vi "subJoystick.vi"(1 "Index":i32=1) -> ()   [LabVIEW 2020]
panel:
  out "AxisZ":i32
  in  "joy button":bool caption="evaluate joystick button"
  in  "Save":bool
  in  "Zone":u32 max=256
  in  "Zzero":u32 caption="Z-Null" max=1023
  in  "Yzero":u32 caption="Y-Null" max=1023
  in  "Xzero":u32 caption="X-Null" max=1023
  in  "SetAcc":bool
  in  "AccZ":i32 caption="Z" min=0
  in  "AccY":i32 caption="Y" min=0
  in  "VelZ":dbl caption="Z, [Hz]" step=0.1 format="%.3f"
  in  "VelY":dbl caption="Y, [Hz]" step=0.1 format="%.3f"
  in  "z3":bool caption="3"
  in  "z2":bool caption="2"
  in  "z1":bool caption="1"
  out "RAcc":bool
  out "RVel":bool
  out "AxisY":i32
  out "AxisX":i32
  in  "AccX":i32 caption="X" min=0
  in  "VelX":dbl caption="X, [Hz]" step=0.1 format="%.3f"
  in  "SetVel":bool
  in  "y3":bool caption="3"
  in  "y2":bool caption="2"
  in  "y1":bool caption="1"
  in  "x3":bool caption="3"
  in  "x2":bool caption="2"
  in  "x1":bool caption="1"
  in  "Set":bool
  in  "Close":bool
  # "Axis X"
  # "Axis Y"
  # "Axis Z"
  # "Joystick speed"
  # "Joystick acceleration"
  # "Joystick settings"
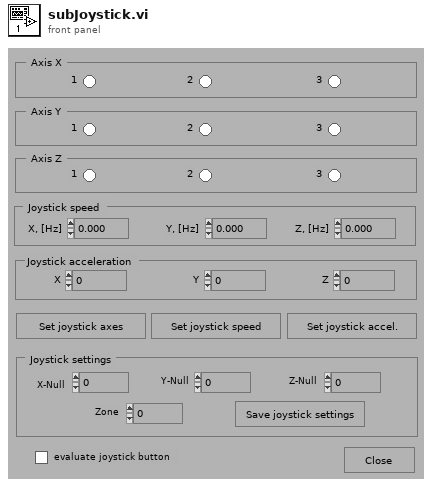
[diagram p1: front panel]
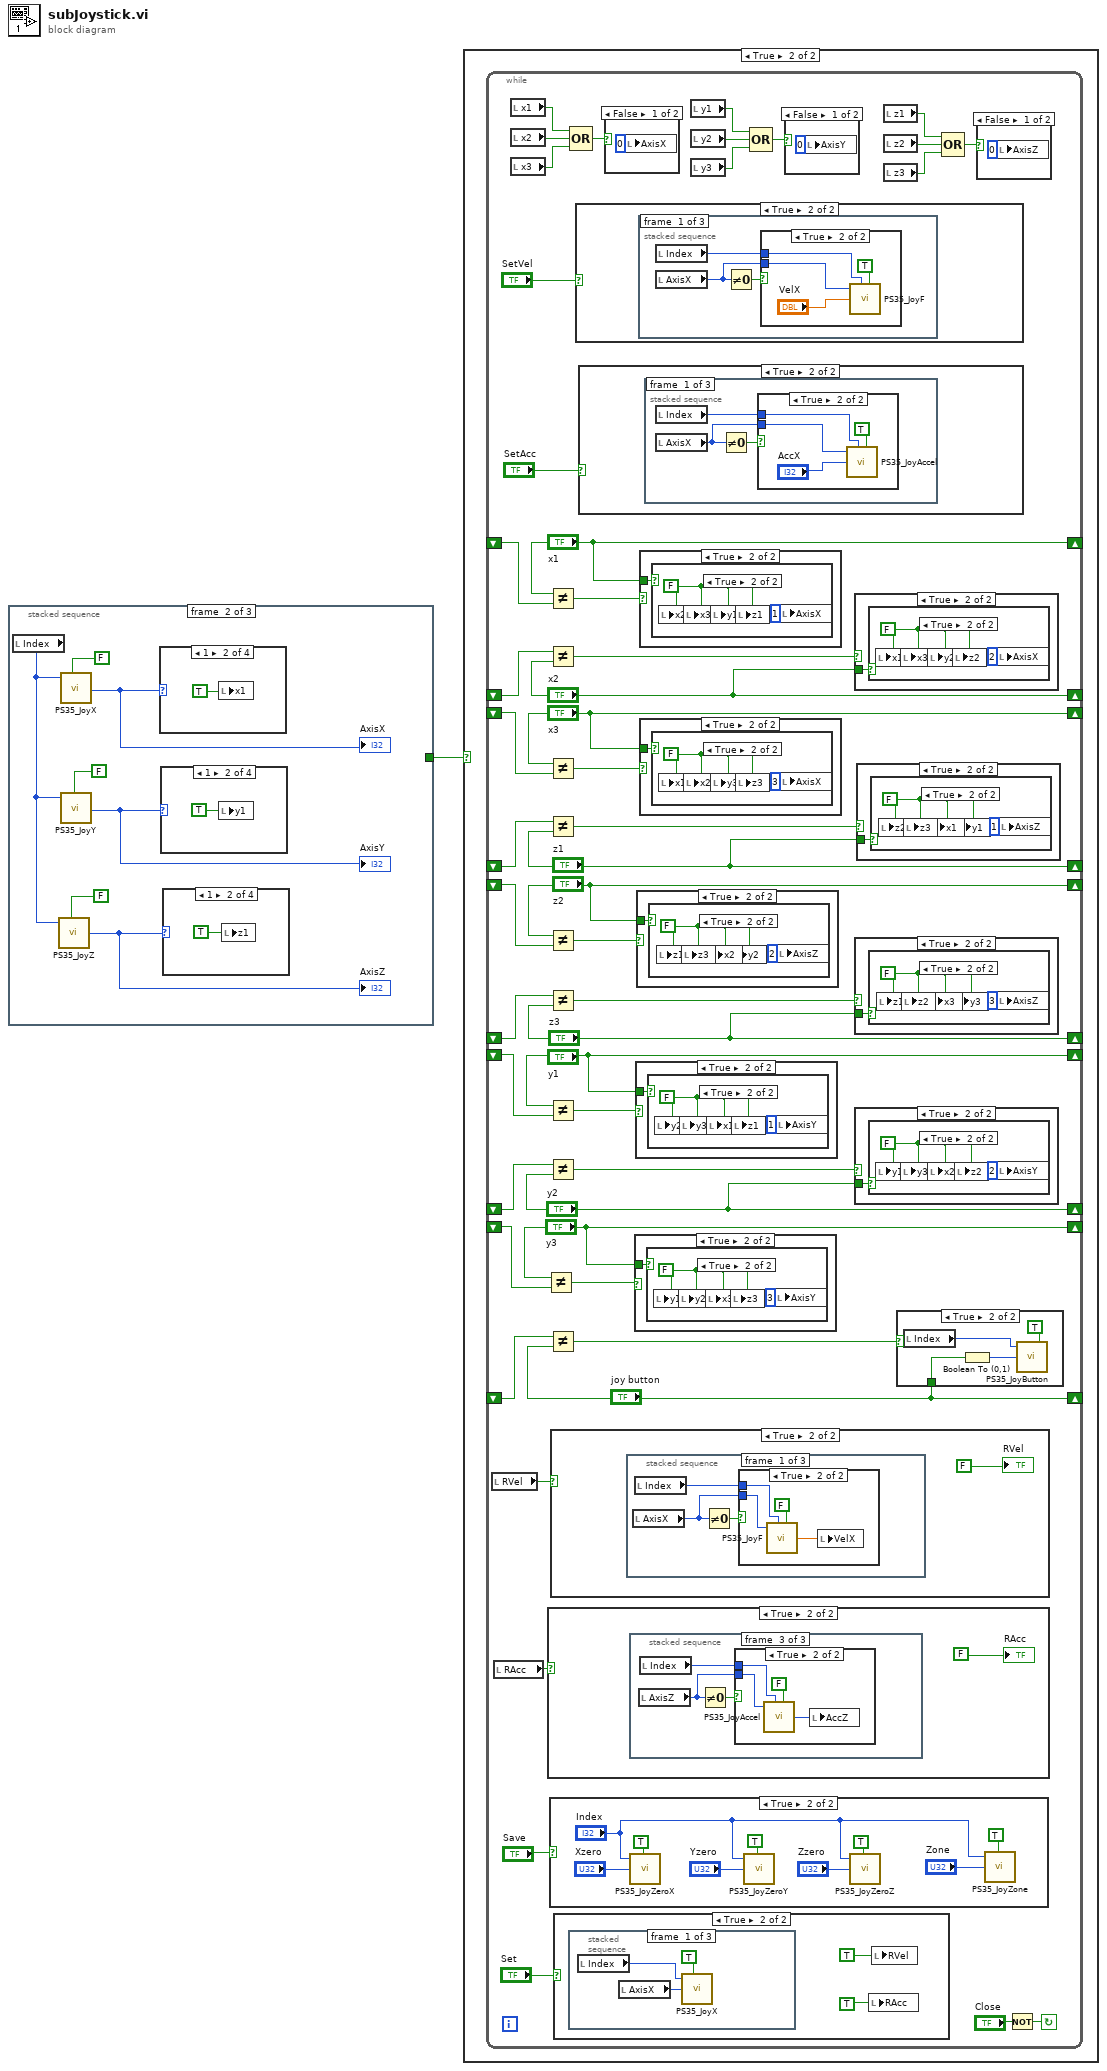
[diagram p0: block diagram]
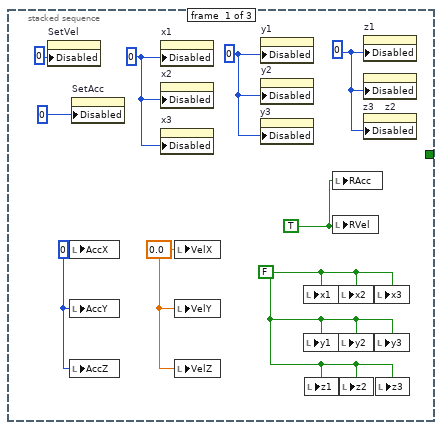
[diagram p2: hidden frame]
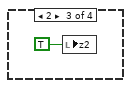
[diagram p4: hidden frame]
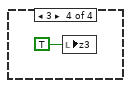
[diagram p5: hidden frame]
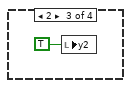
[diagram p7: hidden frame]
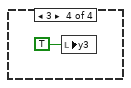
[diagram p8: hidden frame]
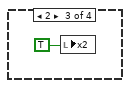
[diagram p10: hidden frame]
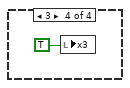
[diagram p11: hidden frame]
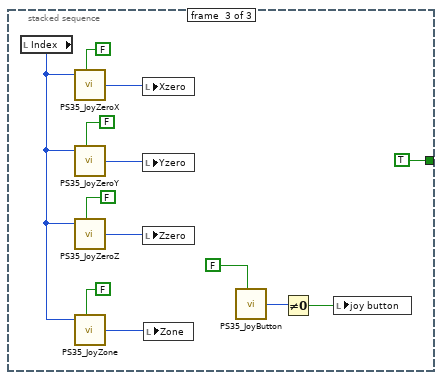
[diagram p12: hidden frame]
diagram:
  n1 = stacked-sequence {
    tunnel: [_ _ TRUE] -> w1
    frame #0 {
      w2 = 0.0 ("VelX")
      w3 = 0 ("AccX")
      w4 = FALSE ("WriteRead")
      w5 = TRUE
      w6 = u8 0 ("Disabled")
      w7 = u8 0 ("Disabled")
      w8 = u8 0 ("Disabled")
      n2 = property on="SetVel" class="Bool"("Disabled"=u8 0) -> ()  [unwired: 2 in, 2 out]
      n3 = local write "AccX"(w3) -> ()
      n4 = local write "AccY"(w3) -> ()
      n5 = local write "AccZ"(w3) -> ()
      n6 = property on="SetAcc" class="Bool"("Disabled"=0 ("Nr")) -> ()  [unwired: 2 in, 2 out]
      n7 = property on="x1" class="Bool (strict)"("Disabled"=w8) -> ()  [unwired: 2 in, 2 out]
      n8 = property on="x2" class="Bool (strict)"("Disabled"=w8) -> ()  [unwired: 2 in, 2 out]
      n9 = property on="x3" class="Bool (strict)"("Disabled"=w8) -> ()  [unwired: 2 in, 2 out]
      n10 = local write "VelX"(w2) -> ()
      n11 = local write "VelY"(w2) -> ()
      n12 = local write "VelZ"(w2) -> ()
      n13 = property on="y1" class="Bool (strict)"("Disabled"=w7) -> ()  [unwired: 2 in, 2 out]
      n14 = property on="y2" class="Bool (strict)"("Disabled"=w7) -> ()  [unwired: 2 in, 2 out]
      n15 = property on="y3" class="Bool (strict)"("Disabled"=w7) -> ()  [unwired: 2 in, 2 out]
      n16 = local write "x1"(w4) -> ()
      n17 = local write "y1"(w4) -> ()
      n18 = local write "z1"(w4) -> ()
      n19 = local write "RAcc"(w5) -> ()
      n20 = local write "RVel"(w5) -> ()
      n21 = local write "x2"(w4) -> ()
      n22 = local write "y2"(w4) -> ()
      n23 = local write "z2"(w4) -> ()
      n24 = property on="z1" class="Bool (strict)"("Disabled"=w6) -> ()  [unwired: 2 in, 2 out]
      n25 = property on="z2" class="Bool (strict)"("Disabled"=w6) -> ()  [unwired: 2 in, 2 out]
      n26 = property on="z3" class="Bool (strict)"("Disabled"=w6) -> ()  [unwired: 2 in, 2 out]
      n27 = local write "x3"(w4) -> ()
      n28 = local write "y3"(w4) -> ()
      n29 = local write "z3"(w4) -> ()
    }
    frame #1 {
      n30 = local read "Index"() -> (w11:i32)
      n31 = call "PS35_JoyZ.vi"("Control unit ID"=w11, "function"=FALSE) -> ("Value-Out"=w12:i32)  [unwired: 6 in, 1 out]
      "AxisZ" <- w12
      n32 = call "PS35_JoyX.vi"("Control unit ID"=w11, "function"=FALSE) -> ("Value-Out"=w14:i32)  [unwired: 6 in, 1 out]
      "AxisX" <- w14
      n33 = call "PS35_JoyY.vi"("Control unit ID"=w11, "function"=FALSE) -> ("Value-Out"=w13:i32)  [unwired: 6 in, 1 out]
      "AxisY" <- w13
      n34 = case shown="1" w14 {
        frame 0, Default {
        }
        frame 1 {
          n35 = local write "x1"(TRUE ("WriteRead")) -> ()
        }
        frame 2 {
          n36 = local write "x2"(TRUE ("WriteRead")) -> ()
        }
        frame 3 {
          n37 = local write "x3"(TRUE ("WriteRead")) -> ()
        }
      }
      n38 = case shown="1" w13 {
        frame 0, Default {
        }
        frame 1 {
          n39 = local write "y1"(TRUE ("y1")) -> ()
        }
        frame 2 {
          n40 = local write "y2"(TRUE ("y1")) -> ()
        }
        frame 3 {
          n41 = local write "y3"(TRUE ("y1")) -> ()
        }
      }
      n42 = case shown="1" w12 {
        frame 0, Default {
        }
        frame 1 {
          n43 = local write "z1"(TRUE ("y1")) -> ()
        }
        frame 2 {
          n44 = local write "z2"(TRUE ("y1")) -> ()
        }
        frame 3 {
          n45 = local write "z3"(TRUE ("y1")) -> ()
        }
      }
    }
    frame #2 {
      n46 = local read "Index"() -> (w27:i32)
      n47 = call "PS35_JoyZeroX.vi"("Control unit ID"=w27, "function"=FALSE) -> ("Value-Out"=w37:i32)  [unwired: 6 in, 1 out]
      n48 = call "PS35_JoyZeroY.vi"("Control unit ID"=w27, "function"=FALSE) -> ("Value-Out"=w36:i32)  [unwired: 6 in, 1 out]
      n49 = call "PS35_JoyZeroZ.vi"("Control unit ID"=w27, "function"=FALSE) -> ("Value-Out"=w33:i32)  [unwired: 6 in, 1 out]
      n50 = call "PS35_JoyZone.vi"("Control unit ID"=w27, "function"=FALSE) -> ("Value-Out"=w32:i32)  [unwired: 6 in, 1 out]
      n51 = local write "Xzero"(w37) -> ()
      n52 = local write "Yzero"(w36) -> ()
      n53 = local write "Zzero"(w33) -> ()
      n54 = local write "Zone"(w32) -> ()
      n55 = call "PS35_JoyButton.vi"("function"=FALSE) -> ("Value-Out"=w29:i32)  [unwired: 7 in, 1 out]
      n56 = Not Equal To 0?(x=w29) -> (x != 0?=w28:bool)
      n57 = local write "joy button"(w28) -> ()
    }
  }
  n58 = case shown="True" w1 {
    frame False {
    }
    frame True {
      n59 = while {
        shift-left: _ -> [w77]
        shift-right: ["joy button"] -> _
        shift-left: _ -> [w79]
        shift-right: ["y3"] -> _
        shift-left: _ -> [w81]
        shift-right: ["y2"] -> _
        shift-left: _ -> [w80]
        shift-right: ["y1"] -> _
        shift-left: _ -> [w82]
        shift-right: ["z3"] -> _
        shift-left: _ -> [w83]
        shift-right: ["z2"] -> _
        shift-left: _ -> [w85]
        shift-right: ["z1"] -> _
        shift-left: _ -> [w84]
        shift-right: ["x3"] -> _
        shift-left: _ -> [w86]
        shift-right: ["x2"] -> _
        shift-left: _ -> [w87]
        shift-right: ["x1"] -> _
        stop <- w89 continue-if-true
        n60 = local read "RVel"() -> (w72:bool)
        n61 = local read "RAcc"() -> (w71:bool)
        n62 = local read "x1"() -> (w50:bool)
        n63 = local read "x2"() -> (w51:bool)
        n64 = local read "x3"() -> (w49:bool)
        n65 = Not Equal?(x="y3", y=w79) -> (x != y?=w53:bool)
        n66 = Not Equal?(x="x1", y=w87) -> (x != y?=w69:bool)
        n67 = Not Equal?(x=w86, y="x2") -> (x != y?=w67:bool)
        n68 = Not Equal?(x="x3", y=w84) -> (x != y?=w65:bool)
        n69 = Not Equal?(x=w85, y="z1") -> (x != y?=w63:bool)
        n70 = Not Equal?(x="z2", y=w83) -> (x != y?=w61:bool)
        n71 = Not Equal?(x=w82, y="z3") -> (x != y?=w59:bool)
        n72 = Not Equal?(x="y1", y=w80) -> (x != y?=w57:bool)
        n73 = Not Equal?(x=w81, y="y2") -> (x != y?=w55:bool)
        n74 = Not Equal?(x=w77, y="joy button") -> (x != y?=w75:bool)
        n75 = case shown="True" w71 {
          frame False {
          }
          frame True {
            n76 = stacked-sequence {
              frame #0 {
                n77 = local read "Index"() -> (w127:i32)
                n78 = local read "AxisX"() -> (w129:i32)
                n79 = Not Equal To 0?(x=w129) -> (x != 0?=w128:bool)
                n80 = case shown="True" w128 {
                  tunnel: w129 -> [_ w133]
                  tunnel: w127 -> [_ w131]
                  frame False {
                    n81 = local write "AccX"(0 ("AccX")) -> ()
                  }
                  frame True {
                    n82 = call "PS35_JoyAccel.vi"("Axis number"=w133, "Control unit ID"=w131, "function"=FALSE ("WriteRead")) -> ("Value-Out"=w132:i32)  [unwired: 5 in, 1 out]
                    n83 = local write "AccX"(w132) -> ()
                  }
                }
              }
              frame #1 {
                n84 = local read "AxisY"() -> (w137:i32)
                n85 = local read "Index"() -> (w135:i32)
                n86 = Not Equal To 0?(x=w137) -> (x != 0?=w136:bool)
                n87 = case shown="True" w136 {
                  tunnel: w137 -> [_ w141]
                  tunnel: w135 -> [_ w139]
                  frame False {
                    n88 = local write "AccY"(0 ("AccX")) -> ()
                  }
                  frame True {
                    n89 = call "PS35_JoyAccel.vi"("Axis number"=w141, "Control unit ID"=w139, "function"=FALSE ("WriteRead")) -> ("Value-Out"=w140:i32)  [unwired: 5 in, 1 out]
                    n90 = local write "AccY"(w140) -> ()
                  }
                }
              }
              frame #2 {
                n91 = local read "AxisZ"() -> (w145:i32)
                n92 = local read "Index"() -> (w143:i32)
                n93 = Not Equal To 0?(x=w145) -> (x != 0?=w144:bool)
                n94 = case shown="True" w144 {
                  tunnel: w145 -> [_ w149]
                  tunnel: w143 -> [_ w147]
                  frame False {
                    n95 = local write "AccZ"(0 ("AccX")) -> ()
                  }
                  frame True {
                    n96 = call "PS35_JoyAccel.vi"("Axis number"=w149, "Control unit ID"=w147, "function"=FALSE ("WriteRead")) -> ("Value-Out"=w148:i32)  [unwired: 5 in, 1 out]
                    n97 = local write "AccZ"(w148) -> ()
                  }
                }
              }
            }
            "RAcc" <- FALSE ("RVel")
          }
        }
        n98 = case shown="True" "Save" {
          frame False {
          }
          frame True {
            n99 = call "PS35_JoyZeroX.vi"("Control unit ID"="Index", "function"=TRUE ("WriteRead"), "Value-In"="Xzero") -> ()  [unwired: 5 in, 2 out]
            n100 = call "PS35_JoyZeroY.vi"("Control unit ID"="Index", "function"=TRUE ("WriteRead"), "Value-In"="Yzero") -> ()  [unwired: 5 in, 2 out]
            n101 = call "PS35_JoyZeroZ.vi"("Control unit ID"="Index", "function"=TRUE ("WriteRead"), "Value-In"="Zzero") -> ()  [unwired: 5 in, 2 out]
            n102 = call "PS35_JoyZone.vi"("Control unit ID"="Index", "function"=TRUE ("WriteRead"), "Value-In"="Zone") -> ()  [unwired: 5 in, 2 out]
          }
        }
        n103 = case shown="True" w72 {
          frame False {
          }
          frame True {
            n104 = stacked-sequence {
              frame #0 {
                n105 = local read "AxisX"() -> (w153:i32)
                n106 = local read "Index"() -> (w152:i32)
                n107 = Not Equal To 0?(x=w153) -> (x != 0?=w154:bool)
                n108 = case shown="True" w154 {
                  tunnel: w153 -> [_ w158]
                  tunnel: w152 -> [_ w156]
                  frame False {
                    n109 = local write "VelX"(0.0 ("VelX")) -> ()
                  }
                  frame True {
                    n110 = call "PS35_JoyF.vi"("Axis number"=w158, "Control unit ID"=w156, "function"=FALSE ("WriteRead")) -> ("dValue-Out"=w157:dbl)  [unwired: 5 in, 1 out]
                    n111 = local write "VelX"(w157) -> ()
                  }
                }
              }
              frame #1 {
                n112 = local read "AxisY"() -> (w161:i32)
                n113 = local read "Index"() -> (w160:i32)
                n114 = Not Equal To 0?(x=w161) -> (x != 0?=w162:bool)
                n115 = case shown="True" w162 {
                  tunnel: w161 -> [_ w166]
                  tunnel: w160 -> [_ w164]
                  frame False {
                    n116 = local write "VelY"(0.0 ("VelX")) -> ()
                  }
                  frame True {
                    n117 = call "PS35_JoyF.vi"("Axis number"=w166, "Control unit ID"=w164, "function"=FALSE ("WriteRead")) -> ("dValue-Out"=w165:dbl)  [unwired: 5 in, 1 out]
                    n118 = local write "VelY"(w165) -> ()
                  }
                }
              }
              frame #2 {
                n119 = local read "Index"() -> (w168:i32)
                n120 = local read "AxisZ"() -> (w169:i32)
                n121 = Not Equal To 0?(x=w169) -> (x != 0?=w170:bool)
                n122 = case shown="True" w170 {
                  tunnel: w169 -> [_ w174]
                  tunnel: w168 -> [_ w172]
                  frame False {
                    n123 = local write "VelZ"(0.0 ("VelX")) -> ()
                  }
                  frame True {
                    n124 = call "PS35_JoyF.vi"("Axis number"=w174, "Control unit ID"=w172, "function"=FALSE ("WriteRead")) -> ("dValue-Out"=w173:dbl)  [unwired: 5 in, 1 out]
                    n125 = local write "VelZ"(w173) -> ()
                  }
                }
              }
            }
            "RVel" <- FALSE ("RVel")
          }
        }
        n126 = case shown="True" "Set" {
          frame False {
          }
          frame True {
            n127 = stacked-sequence {
              frame #0 {
                n128 = local read "Index"() -> (w224:i32)
                n129 = local read "AxisX"() -> (w226:i32)
                n130 = call "PS35_JoyX.vi"("Control unit ID"=w224, "function"=TRUE ("WriteRead"), "Value-In"=w226) -> ()  [unwired: 5 in, 2 out]
              }
              frame #1 {
                n131 = local read "Index"() -> (w227:i32)
                n132 = local read "AxisY"() -> (w229:i32)
                n133 = call "PS35_JoyY.vi"("Control unit ID"=w227, "function"=TRUE ("WriteRead"), "Value-In"=w229) -> ()  [unwired: 5 in, 2 out]
              }
              frame #2 {
                n134 = local read "Index"() -> (w230:i32)
                n135 = local read "AxisZ"() -> (w232:i32)
                n136 = call "PS35_JoyZ.vi"("Control unit ID"=w230, "function"=TRUE ("WriteRead"), "Value-In"=w232) -> ()  [unwired: 5 in, 2 out]
              }
            }
            n137 = local write "RAcc"(TRUE ("WriteRead")) -> ()
            n138 = local write "RVel"(TRUE ("WriteRead")) -> ()
          }
        }
        n139 = Compound Arithmetic op=OR(w50, w51, w49) -> (w48:bool)
        n140 = case shown="True" "SetVel" {
          frame False {
          }
          frame True {
            n141 = stacked-sequence {
              frame #0 {
                n142 = local read "Index"() -> (w201:i32)
                n143 = local read "AxisX"() -> (w202:i32)
                n144 = Not Equal To 0?(x=w202) -> (x != 0?=w203:bool)
                n145 = case shown="True" w203 {
                  tunnel: w202 -> [_ w205]
                  tunnel: w201 -> [_ w204]
                  frame False {
                  }
                  frame True {
                    n146 = call "PS35_JoyF.vi"("Axis number"=w205, "Control unit ID"=w204, "dValue-In"="VelX", "function"=TRUE ("WriteRead")) -> ()  [unwired: 4 in, 2 out]
                  }
                }
              }
              frame #1 {
                n147 = local read "AxisY"() -> (w209:i32)
                n148 = local read "Index"() -> (w208:i32)
                n149 = Not Equal To 0?(x=w209) -> (x != 0?=w210:bool)
                n150 = case shown="True" w210 {
                  tunnel: w209 -> [_ w213]
                  tunnel: w208 -> [_ w211]
                  frame False {
                  }
                  frame True {
                    n151 = call "PS35_JoyF.vi"("Axis number"=w213, "Control unit ID"=w211, "dValue-In"="VelY", "function"=TRUE ("WriteRead")) -> ()  [unwired: 4 in, 2 out]
                  }
                }
              }
              frame #2 {
                n152 = local read "AxisZ"() -> (w216:i32)
                n153 = local read "Index"() -> (w215:i32)
                n154 = Not Equal To 0?(x=w216) -> (x != 0?=w217:bool)
                n155 = case shown="True" w217 {
                  tunnel: w216 -> [_ w220]
                  tunnel: w215 -> [_ w218]
                  frame False {
                  }
                  frame True {
                    n156 = call "PS35_JoyF.vi"("Axis number"=w220, "Control unit ID"=w218, "dValue-In"="VelZ", "function"=TRUE ("WriteRead")) -> ()  [unwired: 4 in, 2 out]
                  }
                }
              }
            }
          }
        }
        n157 = case shown="True" "SetAcc" {
          frame False {
          }
          frame True {
            n158 = stacked-sequence {
              frame #0 {
                n159 = local read "Index"() -> (w176:i32)
                n160 = local read "AxisX"() -> (w178:i32)
                n161 = Not Equal To 0?(x=w178) -> (x != 0?=w177:bool)
                n162 = case shown="True" w177 {
                  tunnel: w178 -> [_ w181]
                  tunnel: w176 -> [_ w179]
                  frame False {
                  }
                  frame True {
                    n163 = call "PS35_JoyAccel.vi"("Axis number"=w181, "Control unit ID"=w179, "Value-In"="AccX", "function"=TRUE ("WriteRead")) -> ()  [unwired: 4 in, 2 out]
                  }
                }
              }
              frame #1 {
                n164 = local read "AxisY"() -> (w185:i32)
                n165 = local read "Index"() -> (w183:i32)
                n166 = Not Equal To 0?(x=w185) -> (x != 0?=w184:bool)
                n167 = case shown="True" w184 {
                  tunnel: w185 -> [_ w188]
                  tunnel: w183 -> [_ w186]
                  frame False {
                  }
                  frame True {
                    n168 = call "PS35_JoyAccel.vi"("Axis number"=w188, "Control unit ID"=w186, "Value-In"="AccY", "function"=TRUE ("WriteRead")) -> ()  [unwired: 4 in, 2 out]
                  }
                }
              }
              frame #2 {
                n169 = local read "AxisZ"() -> (w192:i32)
                n170 = local read "Index"() -> (w190:i32)
                n171 = Not Equal To 0?(x=w192) -> (x != 0?=w191:bool)
                n172 = case shown="True" w191 {
                  tunnel: w192 -> [_ w195]
                  tunnel: w190 -> [_ w193]
                  frame False {
                  }
                  frame True {
                    n173 = call "PS35_JoyAccel.vi"("Axis number"=w195, "Control unit ID"=w193, "Value-In"="AccZ", "function"=TRUE ("WriteRead")) -> ()  [unwired: 4 in, 2 out]
                  }
                }
              }
            }
          }
        }
        n174 = case shown="False" w48 {
          frame False {
            n175 = local write "AxisX"(0 ("Disabled")) -> ()
          }
          frame True {
          }
        }
        n176 = case shown="True" w53 {
          tunnel: "y3" -> [_ w93]
          frame False {
          }
          frame True {
            n177 = case shown="True" w93 {
              frame False {
              }
              frame True {
                w94 = FALSE
                n178 = local write "y1"(w94) -> ()
                n179 = local write "y2"(w94) -> ()
                n180 = local write "x3"(w94) -> ()
                n181 = local write "z3"(w94) -> ()
                n182 = local write "AxisY"(3 ("Disabled")) -> ()
              }
            }
          }
        }
        n183 = case shown="True" w57 {
          tunnel: "y1" -> [_ w99]
          frame False {
          }
          frame True {
            n184 = case shown="True" w99 {
              frame False {
              }
              frame True {
                w100 = FALSE
                n185 = local write "y2"(w100) -> ()
                n186 = local write "y3"(w100) -> ()
                n187 = local write "x1"(w100) -> ()
                n188 = local write "z1"(w100) -> ()
                n189 = local write "AxisY"(1 ("Disabled")) -> ()
              }
            }
          }
        }
        n190 = case shown="True" w61 {
          tunnel: "z2" -> [_ w105]
          frame False {
          }
          frame True {
            n191 = case shown="True" w105 {
              frame False {
              }
              frame True {
                w106 = FALSE
                n192 = local write "z1"(w106) -> ()
                n193 = local write "z3"(w106) -> ()
                n194 = local write "x2"(w106) -> ()
                n195 = local write "y2"(w106) -> ()
                n196 = local write "AxisZ"(2 ("Disabled")) -> ()
              }
            }
          }
        }
        n197 = case shown="True" w69 {
          tunnel: "x1" -> [_ w233]
          frame False {
          }
          frame True {
            n198 = case shown="True" w233 {
              frame False {
              }
              frame True {
                w235 = FALSE
                n199 = local write "x2"(w235) -> ()
                n200 = local write "x3"(w235) -> ()
                n201 = local write "y1"(w235) -> ()
                n202 = local write "z1"(w235) -> ()
                n203 = local write "AxisX"(1 ("Disabled")) -> ()
              }
            }
          }
        }
        n204 = case shown="True" w65 {
          tunnel: "x3" -> [_ w111]
          frame False {
          }
          frame True {
            n205 = case shown="True" w111 {
              frame False {
              }
              frame True {
                w112 = FALSE
                n206 = local write "x1"(w112) -> ()
                n207 = local write "x2"(w112) -> ()
                n208 = local write "y3"(w112) -> ()
                n209 = local write "z3"(w112) -> ()
                n210 = local write "AxisX"(3 ("Disabled")) -> ()
              }
            }
          }
        }
        n211 = local read "y1"() -> (w45:bool)
        n212 = local read "y2"() -> (w44:bool)
        n213 = local read "y3"() -> (w46:bool)
        n214 = Compound Arithmetic op=OR(w45, w44, w46) -> (w47:bool)
        n215 = case shown="False" w47 {
          frame False {
            n216 = local write "AxisY"(0 ("Disabled")) -> ()
          }
          frame True {
          }
        }
        n217 = case shown="True" w67 {
          tunnel: "x2" -> [_ w114]
          frame False {
          }
          frame True {
            n218 = case shown="True" w114 {
              frame False {
              }
              frame True {
                w115 = FALSE
                n219 = local write "x1"(w115) -> ()
                n220 = local write "x3"(w115) -> ()
                n221 = local write "y2"(w115) -> ()
                n222 = local write "z2"(w115) -> ()
                n223 = local write "AxisX"(2 ("Disabled")) -> ()
              }
            }
          }
        }
        n224 = case shown="True" w59 {
          tunnel: "z3" -> [_ w102]
          frame False {
          }
          frame True {
            n225 = case shown="True" w102 {
              frame False {
              }
              frame True {
                w103 = FALSE
                n226 = local write "z1"(w103) -> ()
                n227 = local write "z2"(w103) -> ()
                n228 = local write "x3"(w103) -> ()
                n229 = local write "y3"(w103) -> ()
                n230 = local write "AxisZ"(3 ("Disabled")) -> ()
              }
            }
          }
        }
        n231 = case shown="True" w55 {
          tunnel: "y2" -> [_ w96]
          frame False {
          }
          frame True {
            n232 = case shown="True" w96 {
              frame False {
              }
              frame True {
                w97 = FALSE
                n233 = local write "y1"(w97) -> ()
                n234 = local write "y3"(w97) -> ()
                n235 = local write "x2"(w97) -> ()
                n236 = local write "z2"(w97) -> ()
                n237 = local write "AxisY"(2 ("Disabled")) -> ()
              }
            }
          }
        }
        n238 = case shown="True" w63 {
          tunnel: "z1" -> [_ w108]
          frame False {
          }
          frame True {
            n239 = case shown="True" w108 {
              frame False {
              }
              frame True {
                w109 = FALSE
                n240 = local write "z2"(w109) -> ()
                n241 = local write "z3"(w109) -> ()
                n242 = local write "x1"(w109) -> ()
                n243 = local write "y1"(w109) -> ()
                n244 = local write "AxisZ"(1 ("Disabled")) -> ()
              }
            }
          }
        }
        n245 = local read "z1"() -> (w42:bool)
        n246 = local read "z2"() -> (w43:bool)
        n247 = local read "z3"() -> (w41:bool)
        n248 = case shown="True" w75 {
          tunnel: "joy button" -> [_ w198]
          frame False {
          }
          frame True {
            n249 = local read "Index"() -> (w197:i32)
            n250 = Boolean To (0,1)(Boolean=w198) -> (0, 1=w199:i16)
            n251 = call "PS35_JoyButton.vi"("Control unit ID"=w197, "function"=TRUE ("WriteRead"), "Value-In"=w199) -> ()  [unwired: 5 in, 2 out]
          }
        }
        n252 = Compound Arithmetic op=OR(w42, w43, w41) -> (w40:bool)
        n253 = case shown="False" w40 {
          frame False {
            n254 = local write "AxisZ"(0 ("Disabled")) -> ()
          }
          frame True {
          }
        }
        n255 = Not(x="Close") -> (.not. x?=w89:bool)
      }
    }
  }
